vi "FOR LOOP=fn.vi"() -> ()   [LabVIEW 2012]
panel:
  out "Array 2":dbl[](array[numeric])
  out "Array":dbl[](array[numeric])
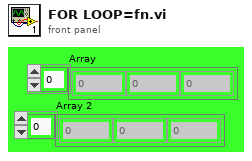
[diagram p1: front panel]
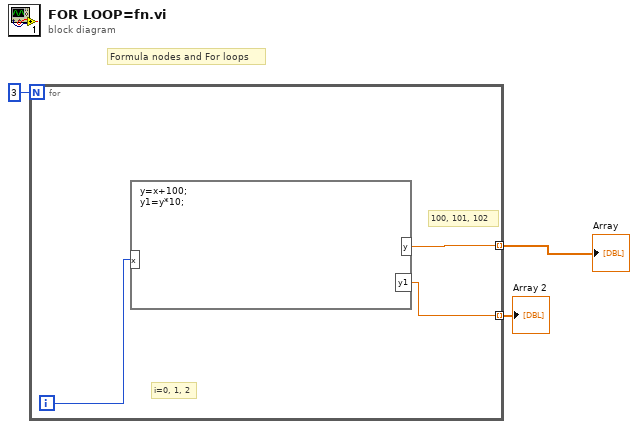
[diagram p0: block diagram]
diagram:
  # "Formula nodes and For loops"
  n1 = for {
    N: 3 -> [_]
    tunnel: [w6] -> w3 mode=indexing
    tunnel: [w4] -> w1 mode=indexing
    i -> [w5]
    # "100, 101, 102"
    # "i=0, 1, 2"
    n2 = formula code="y=x+100;\ny1=y*10;"("x"=w5) -> ("y"=w6:dbl, "y1"=w4:dbl)
  }
  "Array" <- w3
  "Array 2" <- w1
